vi "Get Error Log Directory Path.vi"() -> (3 "Error Log Path":path)   [LabVIEW 2020, in "Utilities.lvlib"]
uses:
  tests/Error Handler Tests/Error Handler Tests.lvclass/Error Handler Tests.ctl
  Utilities.lvlib
  <vilib>/Utility/sysdir.llb/System Directory Type.ctl
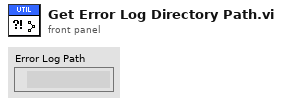
[diagram p1: front panel]
types:
  T1 = typedef "System Directory Type.ctl" = i32
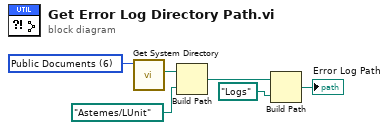
[diagram p0: block diagram]
diagram:
  w1 = T1 6 items=["User Home"=0, "User Desktop"=1, "User Documents"=2, "User Application Data"=3, "User Preferences"=4, "User Temporary"=5, "Public Documents"=6, "Public Application Data"=7, "Public Preferences"=8, "Public Cache"=13, "System Core Libraries"=9, "System Installed Libraries"=10, "Application Files"=11, "Boot Volume Root"=12] ("system directory type")
  n1 = call <vilib>:"Get System Directory.vi"("system directory type"=w1) -> ("system directory"=w3:path)  [unwired: 10 in]
  n2 = Build Path(base path=w3, name or relative path=path "Astemes/LUnit") -> (appended path=w4:path)
  n3 = Build Path(base path=w4, name or relative path=path "Logs") -> (appended path=→"Error Log Path":path)
